vi "Create New PPL Extension.vi"(0 "project refnum":refnum<vi>, 5 "build specification name":string, 11 "error in (no error)":errorcluster) -> (4 "NI_AB_API_Build out":refnum<class "NI_AB_API_PPL_Extensions.lvclass">, 15 "error out":errorcluster)   [LabVIEW 2021, in "NI_AB_API_PPL_Extensions.lvclass"]
uses:
  NI_AB_API_PPL_Extensions.lvclass
  C:/Program Files/National Instruments/LabVIEW 2021/vi.lib/AppBuilder/AB_API/Build/NI_AB_API_Build.lvclass
  <vilib>/AppBuilder/AB_API/common/AB_API Build Object Type.ctl
  <vilib>/AppBuilder/AB_Classes/PackedLib/AB_PackedLibrary.lvclass
  C:/Program Files/National Instruments/LabVIEW 2021/vi.lib/AppBuilder/AB_Classes/Build/AB_Build.lvclass
  NI_AB_API_PPL_Extensions.lvclass/NI_AB_API_PPL_Extensions.ctl
  <vilib>/AppBuilder/AB_API/Build/NI_AB_API_Build.lvclass
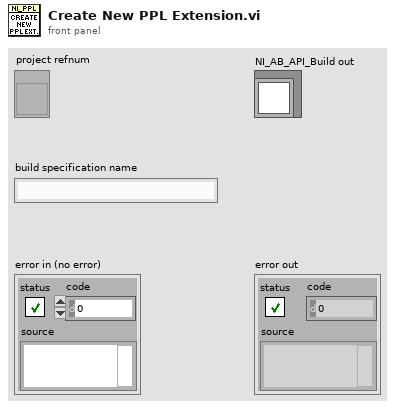
[diagram p1: front panel]
types:
  T1 = typedef "AB_API Build Object Type.ctl" = enum16{"Source Distribution", "DLL", "EXE", "Installer", "Zip File", "RESTful WS", "RTEXE", "Packed Library", "C Generation ", ".NET Interop Assembly"}
  T2 = typedef "ItemRef.ctl" = u64
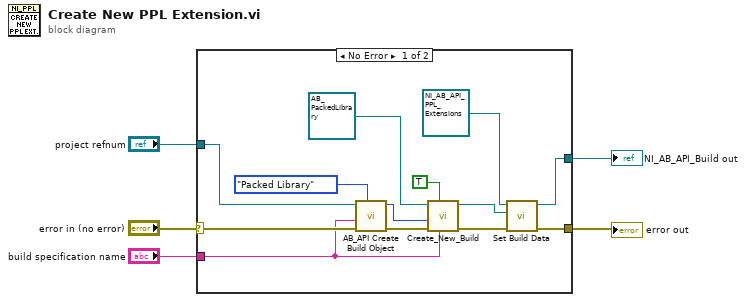
[diagram p0: block diagram]
diagram:
  n1 = case shown="No Error" "error in (no error)" {
    selector: "error in (no error)" -> [w17 w19]
    tunnel: [w16 w19] -> w5
    tunnel: "project refnum" -> [w14 _]
    tunnel: "build specification name" -> [w8 _]
    tunnel: [w15 _] -> w1
    frame No Error {
      n2 = call <vilib>:"AB_API Create Build Object.vi"("Build object type"=AB_API_Build_Object_Type."Packed Library", "error in (no error)"=w17, "Build spec name"=w8, "Project Refnum"=w14) -> ("error out"=w12:errorcluster, "Build object"=w11:T2)  [unwired: 1 in, 5 out]
      n3 = call-dynamic "Create_New_Build.vi"("buildSpecName"=w8, "Programmatic? (false)"=TRUE, "error in (no error)"=w12, "buildObject"=w11, "AB_PackedLibrary in"=refnum<class "AB_PackedLibrary.lvclass"> refnum) -> ("error out"=w9:errorcluster, "AB_PackedLibrary out"=w10:refnum<class "AB_PackedLibrary.lvclass">)  [unwired: 5 in]
      n4 = call <vilib>:"Set Build Data.vi"("error in (no error)"=w9, "AB_Build.lvclass"=w10, "NI_AB_API_Build in"=refnum<class "NI_AB_API_PPL_Extensions.lvclass"> refnum ("NI_AB_API_PPL_Extensions.lvclass")) -> ("error out"=w16:errorcluster, "NI_AB_API_Build out"=w15:refnum<class "NI_AB_API_PPL_Extensions.lvclass">)  [unwired: 7 in]
    }
    frame Error {
    }
  }
  "error out" <- w5
  "NI_AB_API_Build out" <- w1
